vi "PixelInterp.vi"(6 "IndexVals":sgl[](array[numeric]), 8 "Array data":dbl[][](array[numeric])) -> (0 "Synth App Out":dbl[][](array[numeric]))   [LabVIEW 2022 SP3]
uses:
  <vilib>/gmath/NI_Gmath.lvlib
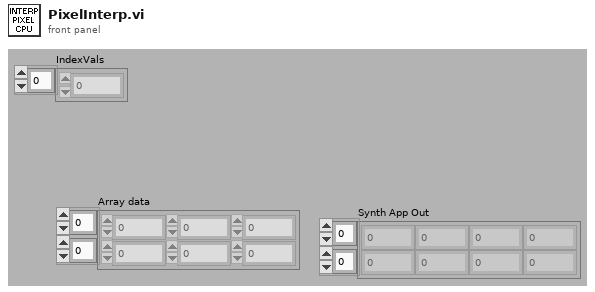
[diagram p1: front panel]
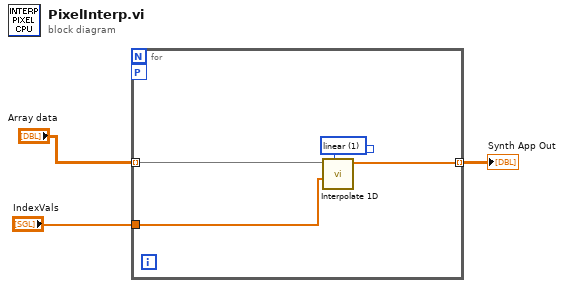
[diagram p0: block diagram]
diagram:
  n1 = for {
    tunnel: "IndexVals" -> [w6]
    tunnel: "Array data" -> [w5] mode=indexing
    tunnel: [w4] -> w1 mode=indexing
    workers-P: _ -> [_]
    w7 = 1 items=["nearest", "linear", "spline", "cubic Hermite", "Lagrange"] ("method")
    n2 = call <vilib>:"Interpolate 1D.vi"("method"=w7, "xi"=w6, "Y"=w5) -> ("yi"=w4:dbl[])  [unwired: 6 in, 2 out]
  }
  "Synth App Out" <- w1
